vi "Equivalence Ratio Math.vi"(1 "Cluster in":T1={"Fuel Flow Rate"=-1.4512315853703328e-05, "Water Flow Rate"=5.644711627352018, "T_in Water"=19.790495447361533, "T_out Water"=21.32835186972947, "Oxygen Flow Rate"=-0.1} {"Oxygen Flow Rate" format="%#_13g"; "T_out Water" format="%#_13g"; "T_in Water" format="%#_13g"; "Water Flow Rate" format="%#_13g"; "Fuel Flow Rate" format="%#_13g"}) -> (0 "Cluster out":cluster{"Phi":dbl, "Q_water":dbl, "Q_fuel":dbl}={"Phi"=0.288245324821388, "Q_water"=605.5550726241157, "Q_fuel"=-12612.943954770637} {"Q_fuel" format="%#_13g"; "Q_water" format="%#_13g"; "Phi" format="%#_13g"})   [LabVIEW 2018]
panel:
  out "m_dot O2":dbl=-0.14285699999999998 format="%#_13g"
  out "m_dot fuel":dbl=-0.01182463495759747 format="%#_13g"
  in  "Stoichiometric Ratio":dbl=0.28716 format="%#_13g"
  in  "Chemical Ptl of Kerosene [J/kg]":dbl=64000000.0 format="%#_13g"
  in  "Density of Kerosene [g/L]":dbl=814.8 format="%#_13g"
  in  "Density of O2 [g/L]":dbl=1.42857 format="%#_13g"
  in  "Alicat Standard P [psi]":dbl=14.696 format="%#_13g"
  in  "Alicat Standard T [K]":dbl=298.15 format="%#_13g"
  in  "Density of Water [kg/L]":dbl=1.0 format="%#_13g"
  in  "Heat Capacity of Water [J/kgC]":dbl=4185.5 format="%#_13g"
  # "Constants"
  # "Outputs"
  # "Input"
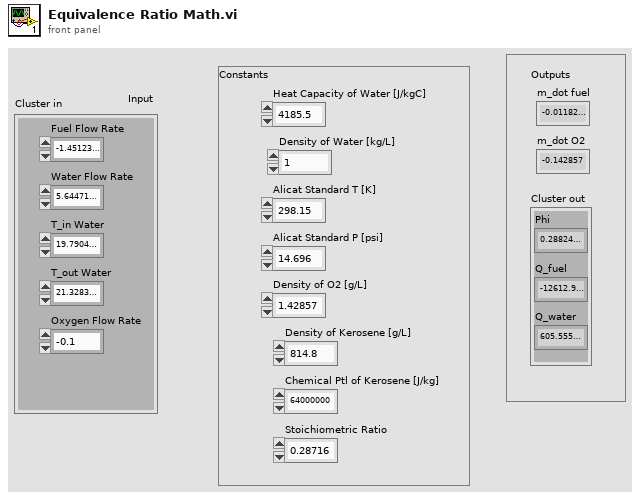
[diagram p1: front panel]
types:
  T1 = cluster{"Fuel Flow Rate":dbl, "Water Flow Rate":dbl, "T_in Water":dbl, "T_out Water":dbl, "Oxygen Flow Rate":dbl}
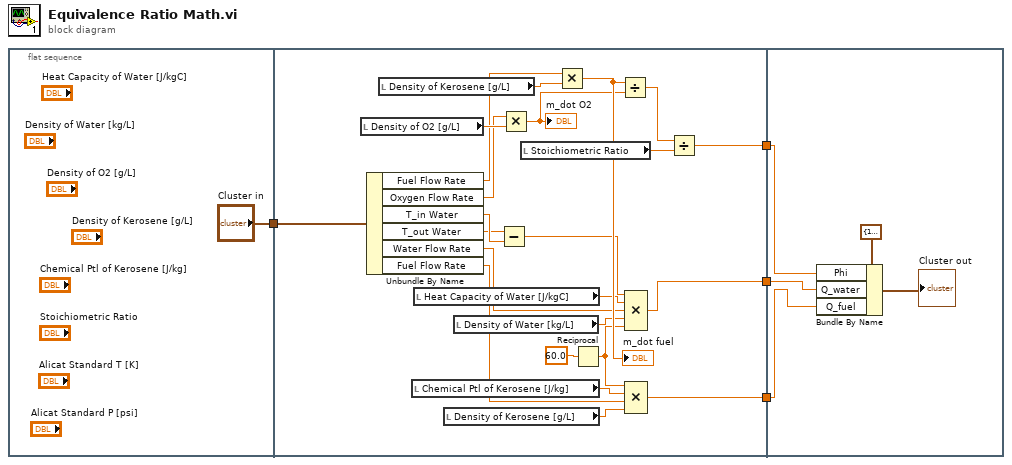
[diagram p0: block diagram]
diagram:
  n1 = flat-sequence {
    tunnel: ["Cluster in"] -> w1
    tunnel: [w15] -> w4
    tunnel: [w14] -> w3
    tunnel: [w13] -> w2
    tunnel: w1 -> [w12]
    tunnel: w4 -> [w33]
    tunnel: w3 -> [w32]
    tunnel: w2 -> [w31]
    frame #0 {
    }
    frame #1 {
      n2 = local read "Density of O2 [g/L]"() -> (w27:dbl)
      n3 = Unbundle By Name(w12) -> ("Fuel Flow Rate"=w11:dbl, "Oxygen Flow Rate"=w10:dbl, "T_in Water"=w9:dbl, "T_out Water"=w8:dbl, "Water Flow Rate"=w7:dbl, "Fuel Flow Rate"=w6:dbl)
      n4 = local read "Density of Kerosene [g/L]"() -> (w28:dbl)
      n5 = local read "Chemical Ptl of Kerosene [J/kg]"() -> (w17:dbl)
      n6 = local read "Heat Capacity of Water [J/kgC]"() -> (w21:dbl)
      n7 = local read "Density of Kerosene [g/L]"() -> (w16:dbl)
      n8 = local read "Density of Water [kg/L]"() -> (w20:dbl)
      n9 = Subtract(x=w8, y=w9) -> (x-y=w22:dbl)
      n10 = Multiply(x=w10, y=w27) -> (x*y=w25:dbl)
      "m_dot O2" <- w25
      n11 = local read "Stoichiometric Ratio"() -> (w23:dbl)
      n12 = Multiply(x=w11, y=w28) -> (x*y=w26:dbl)
      "m_dot fuel" <- w26
      n13 = Reciprocal(x=60.0 ("value")) -> (1/x=w18:dbl)
      n14 = Divide(x=w26, y=w25) -> (x/y=w24:dbl)
      n15 = Compound Arithmetic op=MULTIPLY(w22, w21, w7, w20, w18) -> (w14:dbl)
      n16 = Compound Arithmetic op=MULTIPLY(w18, w17, w6, w16) -> (w13:dbl)
      n17 = Divide(x=w24, y=w23) -> (x/y=w15:dbl)
    }
    frame #2 {
      n18 = Bundle By Name(cluster=cluster{"Phi":dbl, "Q_water":dbl, "Q_fuel":dbl} {"Phi"=1.6357098716730532, "Q_water"=103.06960046365045, "Q_fuel"=-71574.85364406662} ("Cluster out 2"), "Phi"=w33, "Q_water"=w32, "Q_fuel"=w31) -> (→"Cluster out":cluster{"Phi":dbl, "Q_water":dbl, "Q_fuel":dbl})
    }
  }
